vi "UHR-Fleezers Control (host) -Leonardo 04-2018 V4_fish.vi"(0 "Tab Green FB":T5(tab)=enum."Trap Control (RF)") -> ()   [LabVIEW 2014] (continued)
          tunnel: [w3580 w3581] -> w3547
          frame False {
          }
          frame True {
            n1861 = Array Subset(array=w3586, index (row)=0 ("index"), length (row)=4 ("length"), index (col)=0 ("index"), length (col)=1 ("length")) -> (w3581:T47)
          }
        }
        n1862 = feedback-in #9(w3547) -> ()
        n1863 = Split 1D Array(array=w3561, index=2) -> (first subarray=→"FFT 1":cluster{"f0":dbl, "df":dbl, "magnitude":dbl[]}[], second subarray=→"FFT 2":cluster{"f0":dbl, "df":dbl, "magnitude":dbl[]}[])
      }
    }
    n1864 = Index Array(array=w2395, index=1) -> (element=w2403:waveform(dbl))
    n1865 = case "For displaying the high resolution display (no downsampling)" shown="True" w2459 {
      tunnel: w2422 -> [_ w2789]
      frame False {
      }
      frame True {
        n1866 = Index Array(array=w2789, index="High Res. Display") -> (element=w2790:waveform(dbl))
        n1867 = call <vilib>:"Std Deviation and Variance.vi"("X"=w2790) -> ("mean"=w2797:dbl, "standard deviation"=w2802:dbl)  [unwired: 1 in, 1 out]
        "Mean Intensity" <- w2797
        "Sigma" <- w2802
        n1868 = Subtract(x=w2790, y=w2797) -> (x-y=w2796:waveform(dbl))
        n1869 = Select(t=w2796, s="Subtract mean", f=w2790) -> (s? t:f=→"1 Channel":waveform(dbl))
        n1870 = Divide(x=w2802, y=w2797) -> (x/y=→"Sigma/Mean":dbl)
        n1871 = feedback #10(1) -> (w2791:i32)
        n1872 = Greater Or Equal?(x=w2791, y="Slow mean N ave.") -> (x >= y?=w2804:bool)
        n1873 = Increment(x=w2791) -> (x+1=w2806:i32)
        n1874 = Select(t=1, s=w2804, f=w2806) -> (s? t:f=w2793:i32)
        n1875 = feedback-in #10(w2793) -> ()
        n1876 = feedback #11() -> (w2794:waveform(dbl))  [unwired: 1 out]
        n1877 = case shown="Default" w2791 {
          tunnel: [w2809 w2812] -> w2795
          tunnel: w2794 -> [w2811 _]
          tunnel: w2790 -> [w2810 w2812]
          frame Default {
            n1878 = call-poly <vilib>:"Append Waveforms.vi"("waveform B"=w2810, "waveform A"=w2811) -> ("waveform out"=w2809:waveform(dbl))  [unwired: 1 in, 8 out]
          }
          frame 1 {
          }
        }
        n1879 = feedback-in #11(w2795) -> ()
        n1880 = case shown="True" w2804 {
          tunnel: w2795 -> [_ w2808]
          frame False {
          }
          frame True {
            n1881 = call-poly <vilib>:"Mean.vi"("X"=w2808) -> ("mean"=→"Slow mean":dbl)  [unwired: 1 out]
          }
        }
      }
    }
    n1882 = case "For plotting results of scanning MCL" shown="True" w2529 {
      tunnel: w2528 -> [_ w2929]
      tunnel: w2452 -> [_ w3025]
      tunnel: w2537 -> [_ _]
      tunnel: w2422 -> [_ w2999]
      tunnel: w2397 -> [_ w2930]
      tunnel: w2396 -> [_ w2903]
      frame False {
      }
      frame True {
        w2910 = u32 0 items=["Horizontal", "Vertical", "Central", "1st Diagonal", "2nd Diagonal"] ("Type of Symmetry")
        w2938 = u32 0 items=["Horizontal", "Vertical", "Central", "1st Diagonal", "2nd Diagonal"] ("Type of Symmetry")
        w2941 = u32 0 items=["Horizontal", "Vertical", "Central", "1st Diagonal", "2nd Diagonal"] ("Type of Symmetry")
        w2970 = u32 0 items=["Horizontal", "Vertical", "Central", "1st Diagonal", "2nd Diagonal"] ("Type of Symmetry")
        n1883 = Index Array(array=w2999, index=10) -> (element=w3005:waveform(dbl))
        n1884 = Index Array(array=w2999, index=11) -> (element=w3002:waveform(dbl))
        n1885 = local read "Cycles/step (MCL)"() -> (w2955:u64)
        n1886 = Index Array(array=w2999, index="Channel") -> (element=w3001:waveform(dbl))
        n1887 = Unbundle(w2903) -> ("New Image"=w2902:T3, "New Image"=w2901:T3, "New Image"=w2900:T3, "New Image"=w2899:T3)
        n1888 = Unbundle By Name(w3005) -> ("Y"=w2957:dbl[])
        n1889 = Unbundle By Name(w3002) -> ("Y"=w2959:dbl[])
        n1890 = Unbundle By Name(w3001) -> ("Y"=w2964:dbl[])
        n1891 = call "downsample 1D array - double.vi"("Ave N"=w2955, "Array In"=w2957) -> ("Array Out"=w2956:dbl[])  [unwired: 1 out]
        n1892 = call "downsample 1D array - double.vi"("Ave N"=w2955, "Array In"=w2959) -> ("Array Out"=w2958:dbl[])  [unwired: 1 out]
        n1893 = call "downsample 1D array - double.vi"("Ave N"=w2955, "Array In"=w2964) -> ("Array Out"=w2963:dbl[])  [unwired: 1 out]
        n1894 = feedback #12(w3025) -> (w3026:dbl[])
        n1895 = Build Array (concatenate)(w3026, w3025) -> (w3007:dbl[])
        n1896 = feedback #13(w2930) -> (w2932:dbl[])
        n1897 = Build Array (concatenate)(w2932, w2930) -> (w2931:dbl[])
        n1898 = local read "Scan steps (MCL)"() -> (w2912:u64)
        n1899 = Select(t=w3025, s=w2929, f=w3007) -> (s? t:f=w3011:dbl[])
        n1900 = feedback-in #12(w3011) -> ()
        n1901 = Select(t=w2930, s=w2929, f=w2931) -> (s? t:f=w2913:dbl[])
        n1902 = feedback-in #13(w2913) -> ()
        n1903 = local read "Scan lines (y)"() -> (w2898:u64)
        n1904 = local read "N APD Samp/step"() -> (w2914:dbl)
        n1905 = feedback #14(w2956) -> (w3013:dbl[])
        n1906 = Build Array (concatenate)(w3013, w2956) -> (w3004:dbl[])
        n1907 = feedback #15(w2963) -> (w3023:dbl[])
        n1908 = Build Array (concatenate)(w3023, w2963) -> (w3022:dbl[])
        n1909 = feedback #16(w2958) -> (w3015:dbl[])
        n1910 = Build Array (concatenate)(w3015, w2958) -> (w3016:dbl[])
        n1911 = Select(t=w2956, s=w2929, f=w3004) -> (s? t:f=w2960:dbl[])
        n1912 = feedback-in #14(w2960) -> ()
        n1913 = Select(t=w2963, s=w2929, f=w3022) -> (s? t:f=w2962:dbl[])
        n1914 = feedback-in #15(w2962) -> ()
        n1915 = Select(t=w2958, s=w2929, f=w3016) -> (s? t:f=w2961:dbl[])
        n1916 = feedback-in #16(w2961) -> ()
        n1917 = Multiply(x=w2912, y=u64 2) -> (x*y=w2897:u64)
        n1918 = call "integrate 1D array interval - double.vi"("Ave N"=w2914, "Array In"=w2913) -> ("Array Out"=w2925:dbl[])  [unwired: 1 out]
        n1919 = call "integrate 1D array interval - double.vi"("Ave N"=w2914, "Array In"=w3011) -> ("Array Out"=w3010:dbl[])  [unwired: 1 out]
        n1920 = Array Size(array=w2925) -> (size(s)=w2926:i32)
        n1921 = Array Size(array=w3010) -> (size(s)=w3012:i32)
        n1922 = Multiply(x=w2898, y=w2897) -> (x*y=w2928:u64)
        n1923 = Multiply(x=w2898, y=w2897) -> (x*y=w3020:u64)
        n1924 = call-poly <vilib>:"Mean.vi"("X"=w2960) -> ("mean"=w2944:dbl)  [unwired: 1 out]
        n1925 = Subtract(x=w2928, y=w2926) -> (x-y=w2919:u64)
        n1926 = call-poly <vilib>:"Mean.vi"("X"=w2962) -> ("mean"=w2949:dbl)  [unwired: 1 out]
        n1927 = call-poly <vilib>:"Mean.vi"("X"=w2961) -> ("mean"=w2947:dbl)  [unwired: 1 out]
        n1928 = call-poly <vilib>:"Mean.vi"("X"=w2925) -> ("mean"=w2916:dbl)  [unwired: 1 out]
        n1929 = Subtract(x=w3020, y=w3012) -> (x-y=w2954:u64)
        n1930 = call-poly <vilib>:"Mean.vi"("X"=w3010) -> ("mean"=w2951:dbl)  [unwired: 1 out]
        n1931 = Initialize Array(1.0 ("element"), w2919) -> (w2915:dbl[])
        n1932 = Initialize Array(1.0 ("element"), w2954) -> (w2945:dbl[])
        n1933 = Multiply(x=w2915, y=w2916) -> (x*y=w2917:dbl[])
        n1934 = Multiply(x=w2945, y=w2947) -> (x*y=w2948:dbl[])
        n1935 = Multiply(x=w2945, y=w2949) -> (x*y=w2950:dbl[])
        n1936 = Multiply(x=w2945, y=w2944) -> (x*y=w2946:dbl[])
        n1937 = Multiply(x=w2945, y=w2951) -> (x*y=w2952:dbl[])
        n1938 = Build Array (concatenate)(w2960, w2946) -> (w3014:dbl[])
        n1939 = Build Array (concatenate)(w2962, w2950) -> (w3018:dbl[])
        n1940 = Build Array (concatenate)(w2961, w2948) -> (w3017:dbl[])
        n1941 = Build Array (concatenate)(w2925, w2917) -> (w2927:dbl[])
        n1942 = Build Array (concatenate)(w3010, w2952) -> (w3019:dbl[])
        n1943 = Reshape Array(w3014, w2898, w2897) -> (w2980:dbl[][])
        n1944 = Reshape Array(w2927, w2898, w2897) -> (w2923:dbl[][])
        n1945 = Reshape Array(w3018, w2898, w2897) -> (w2972:dbl[][])
        n1946 = Reshape Array(w3017, w2898, w2897) -> (w2987:dbl[][])
        n1947 = Reshape Array(w3019, w2898, w2897) -> (w2997:dbl[][])
        n1948 = Array Subset(array=w2987, index (col)=0 ("index"), length (col)=w2912) -> (w2992:dbl[][])  [unwired: 2 in]
        n1949 = Array Subset(array=w2987, index (col)=w2912) -> (w2990:dbl[][])  [unwired: 3 in]
        n1950 = Array Subset(array=w2972, index (col)=0 ("index"), length (col)=w2912) -> (w2978:dbl[][])  [unwired: 2 in]
        n1951 = Array Subset(array=w2972, index (col)=w2912) -> (w2976:dbl[][])  [unwired: 3 in]
        n1952 = Array Subset(array=w2923, index (col)=0 ("index"), length (col)=w2912) -> (w2922:dbl[][])  [unwired: 2 in]
        n1953 = Array Subset(array=w2923, index (col)=w2912) -> (w2920:dbl[][])  [unwired: 3 in]
        n1954 = Array Subset(array=w2997, index (col)=0 ("index"), length (col)=w2912) -> (w2996:dbl[][])  [unwired: 2 in]
        n1955 = Array Subset(array=w2997, index (col)=w2912) -> (w2994:dbl[][])  [unwired: 3 in]
        n1956 = Array Subset(array=w2980, index (col)=0 ("index"), length (col)=w2912) -> (w2985:dbl[][])  [unwired: 2 in]
        n1957 = Array Subset(array=w2980, index (col)=w2912) -> (w2983:dbl[][])  [unwired: 3 in]
        n1958 = for {
          tunnel: w2992 -> [w3034] mode=indexing
          tunnel: [w3033] -> w2991 mode=indexing
          workers-P: _ -> [_]
          n1959 = Reverse 1D Array(array=w3034) -> (reversed array=w3033:dbl[])
        }
        n1960 = for {
          tunnel: w2978 -> [w3030] mode=indexing
          tunnel: [w3029] -> w2977 mode=indexing
          workers-P: _ -> [_]
          n1961 = Reverse 1D Array(array=w3030) -> (reversed array=w3029:dbl[])
        }
        n1962 = for {
          tunnel: w2922 -> [w3028] mode=indexing
          tunnel: [w3027] -> w2921 mode=indexing
          workers-P: _ -> [_]
          n1963 = Reverse 1D Array(array=w3028) -> (reversed array=w3027:dbl[])
        }
        n1964 = for {
          tunnel: w2996 -> [w3036] mode=indexing
          tunnel: [w3035] -> w2995 mode=indexing
          workers-P: _ -> [_]
          n1965 = Reverse 1D Array(array=w3036) -> (reversed array=w3035:dbl[])
        }
        n1966 = for {
          tunnel: w2985 -> [w3032] mode=indexing
          tunnel: [w3031] -> w2984 mode=indexing
          workers-P: _ -> [_]
          n1967 = Reverse 1D Array(array=w3032) -> (reversed array=w3031:dbl[])
        }
        n1968 = Index Array(array=w2997, index (row)=0) -> (element=→"Waveform Graph":dbl[])  [unwired: 1 in]
        n1969 = Add(x=w2991, y=w2990) -> (x+y=w2989:dbl[][])
        n1970 = Add(x=w2977, y=w2976) -> (x+y=w2975:dbl[][])
        n1971 = Add(x=w2921, y=w2920) -> (x+y=w2905:dbl[][])
        n1972 = Add(x=w2995, y=w2994) -> (x+y=w2969:dbl[][])
        n1973 = Add(x=w2984, y=w2983) -> (x+y=w2982:dbl[][])
        n1974 = Divide(x=w2975, y=2) -> (x/y=w2973:dbl[][])
        n1975 = Divide(x=w2989, y=2) -> (x/y=w2934:dbl[][])
        n1976 = Divide(x=w2982, y=2) -> (x/y=w2936:dbl[][])
        n1977 = To Single Precision Float(number=w2969) -> (single precision float=w2968:sgl[][])
        n1978 = Transpose 2D Array(2D array=w2973) -> (transposed array=→"Data map":dbl[][])
        n1979 = To Single Precision Float(number=w2905) -> (single precision float=w2909:sgl[][])
        n1980 = To Single Precision Float(number=w2934) -> (single precision float=w2940:sgl[][])
        n1981 = To Single Precision Float(number=w2936) -> (single precision float=w2937:sgl[][])
        n1982 = call "IMAQ ArrayToImage"("Image Pixels (Float)"=w2968, "Image"=w2902) -> ("Image Out"=w2971:T3)  [unwired: 8 in, 1 out]
        n1983 = call "IMAQ ArrayToImage"("Image Pixels (Float)"=w2909, "Image"=w2901) -> ("Image Out"=w2911:T3)  [unwired: 8 in, 1 out]
        n1984 = call "IMAQ ArrayToImage"("Image Pixels (Float)"=w2940, "Image"=w2900) -> ("Image Out"=w2942:T3)  [unwired: 8 in, 1 out]
        n1985 = call "IMAQ ArrayToImage"("Image Pixels (Float)"=w2937, "Image"=w2899) -> ("Image Out"=w2939:T3)  [unwired: 8 in, 1 out]
        n1986 = call "IMAQ Symmetry"("Type of Symmetry"=w2970, "Image Src"=w2971) -> ("Image Dst Out"=w2966:T3)  [unwired: 3 in, 1 out]
        n1987 = call "IMAQ Symmetry"("Type of Symmetry"=w2910, "Image Src"=w2911) -> ("Image Dst Out"=w2907:T3)  [unwired: 3 in, 1 out]
        n1988 = call "IMAQ Symmetry"("Type of Symmetry"=w2941, "Image Src"=w2942) -> ("Image Dst Out"=→"Detection Laser X":T3)  [unwired: 3 in, 1 out]
        n1989 = call "IMAQ Symmetry"("Type of Symmetry"=w2938, "Image Src"=w2939) -> ("Image Dst Out"=→"Detection Laser Y":T3)  [unwired: 3 in, 1 out]
        n1990 = call "IMAQ Set Simple Calibration"("Calibration Axis Info"=T37 {"Origin Pixel"={"X"=0.0, "Y"=0.0}, "Angle Relative to Horizontal (deg)"=0.0, "Axis Reference"=0}, "Grid Descriptor"=T38 {"X Step"=0.3, "Y Step"=0.3, "Unit"=enum."Undefined"}, "Image"=w2966) -> ("Calibrated Image"=→"APD 1":T3)  [unwired: 7 in, 1 out]
        n1991 = call "IMAQ Set Simple Calibration"("Calibration Axis Info"=T37 {"Origin Pixel"={"X"=0.0, "Y"=0.0}, "Angle Relative to Horizontal (deg)"=0.0, "Axis Reference"=0}, "Grid Descriptor"=T38 {"X Step"=0.3, "Y Step"=0.3, "Unit"=enum."Undefined"}, "Image"=w2907) -> ("Calibrated Image"=→"APD 2":T3)  [unwired: 7 in, 1 out]
      }
    }
    n1992 = Subtract(x=w2403, y="APD 2 Offset") -> (x-y=w2400:waveform(dbl))
    n1993 = Subtract(x=w2405, y="APD 1 Offset") -> (x-y=w2401:waveform(dbl))
    n1994 = Index Array(array=w2420, index=3) -> (element=w2479:waveform(dbl))
    n1995 = Index Array(array=w2420, index=6) -> (element=w2476:waveform(dbl))
    n1996 = Build Array(w2401, w2400) -> (→"APD Chart":waveform(dbl)[])
    n1997 = Array Size(array=w2469) -> (size(s)=w2517:i32)
    n1998 = call <vilib>:"Std Deviation and Variance.vi"("X"=w2413) -> ("standard deviation"=w2412:dbl)  [unwired: 1 in, 2 out]
    n1999 = Add Array Elements(numeric array=w2413) -> (sum=w2415:u32)
    n2000 = Add Array Elements(numeric array=w2469) -> (sum=w2527:u32)
    n2001 = call <vilib>:"Std Deviation and Variance.vi"("X"=w2469) -> ("standard deviation"=w2468:dbl)  [unwired: 1 in, 2 out]
    n2002 = Divide(x=w2412, y=w2411) -> (x/y=w2408:dbl)
    "Rate sigma (Hz) 2" <- w2408
    n2003 = Multiply(x=w2411, y=w2517) -> (x*y=w2414:dbl)
    "Int. Time (s)" <- w2414
    n2004 = Divide(x=w2415, y=w2414) -> (x/y=w2409:dbl)
    "APD 2 Rate (Hz)" <- w2409
    n2005 = Divide(x=w2527, y=w2414) -> (x/y=w2466:dbl)
    "APD 1 Rate (Hz)" <- w2466
    n2006 = Divide(x=w2468, y=w2411) -> (x/y=w2467:dbl)
    "Rate sigma (Hz)" <- w2467
    n2007 = Divide(x=w2408, y=w2409) -> (x/y=→"Sigma/Mean 2":dbl)
    n2008 = Divide(x=w2467, y=w2466) -> (x/y=→"Sigma/Mean":dbl)
    n2009 = case shown="2" "Calibration" {
      tunnel: "T1 alpha_x (nm/V)" -> [_ w2865 w2886]
      tunnel: "T1 kappa_x (pN/nm)" -> [_ _ w2876]
      tunnel: "T2 alpha_x (nm/V)" -> [_ w2864 w2884]
      tunnel: "T2 kappa_x (pN/nm)" -> [_ _ w2877]
      tunnel: w2479 -> [w2847 w2862 w2882]
      tunnel: w2476 -> [w2846 w2860 w2880]
      tunnel: [w2847 w2859 w2879] -> w2270
      tunnel: [w2846 w2858 w2878] -> w2276
      tunnel: ["T1 X (V)" ("Label.Text") "T1 X (nm)" ("Label.Text") "T1 X (pN)" ("Label.Text")] -> w2497
      tunnel: ["T2 X (V)" ("Label.Text") "T2 X (nm)" ("Label.Text") "T2 X (pN)" ("Label.Text")] -> w2496
      tunnel: ["Position (V)" ("Label.Text") "Position (nm)" ("Label.Text") "Force (pN)" ("Label.Text")] -> w2498
      tunnel: w2478 -> [_ w2850 w2869]
      tunnel: w2480 -> [_ w2853 w2871]
      tunnel: ["Mean (V)" ("Label.Text") "Mean (nm)" ("Label.Text") "Mean (pN)" ("Label.Text")] -> w2493
      tunnel: ["Difference (V)" ("Label.Text") "Difference (nm)" ("Label.Text") "Difference (pN)" ("Label.Text")] -> w2428
      frame 0, Default {
      }
      frame 1 {
        # "position"
        n2010 = Unbundle By Name(w2862) -> ("Y"=w2866:dbl[])
        n2011 = Unbundle By Name(w2860) -> ("Y"=w2851:dbl[])
        n2012 = Subtract(x=w2866, y=w2853) -> (x-y=w2854:dbl[])
        n2013 = Subtract(x=w2851, y=w2850) -> (x-y=w2852:dbl[])
        n2014 = Multiply(x=w2852, y=w2864) -> (x*y=w2861:dbl[])
        n2015 = Multiply(x=w2865, y=w2854) -> (x*y=w2863:dbl[])
        n2016 = Bundle By Name(cluster=w2860, "Y"=w2861) -> (w2858:waveform(dbl))
        n2017 = Bundle By Name(cluster=w2862, "Y"=w2863) -> (w2859:waveform(dbl))
      }
      frame 2 {
        # "force"
        n2018 = Unbundle By Name(w2882) -> ("Y"=w2887:dbl[])
        n2019 = Unbundle By Name(w2880) -> ("Y"=w2885:dbl[])
        n2020 = Subtract(x=w2885, y=w2869) -> (x-y=w2870:dbl[])
        n2021 = Subtract(x=w2887, y=w2871) -> (x-y=w2872:dbl[])
        n2022 = Compound Arithmetic op=MULTIPLY(w2870, w2884, w2877) -> (w2881:dbl[])
        n2023 = Compound Arithmetic op=MULTIPLY(w2876, w2886, w2872) -> (w2883:dbl[])
        n2024 = Bundle By Name(cluster=w2880, "Y"=w2881) -> (w2878:waveform(dbl))
        n2025 = Bundle By Name(cluster=w2882, "Y"=w2883) -> (w2879:waveform(dbl))
      }
    }
    n2026 = feedback-in #17("Calibration") -> ()
    n2027 = feedback #17(u16 1 ("Calibration")) -> (w2500:u16)
    n2028 = local read "Trap 2 Bead Size (nm)"() -> (w2308:dbl)
    n2029 = local read "Trap 1 Bead Size (nm)"() -> (w2307:dbl)
    n2030 = local read "AOM X Cal (nm/MHz)"() -> (w2305:dbl)
    n2031 = local read "Trap Delta (MHz)"() -> (w2304:dbl)
    n2032 = Not Equal?(x=w2500, y="Calibration") -> (x != y?=w2457:bool)
    n2033 = Multiply(x=w2305, y=w2304) -> (x*y=w2309:dbl)
    n2034 = Unbundle By Name(w2270) -> ("Y"=w2275:dbl[])
    n2035 = Unbundle By Name(w2276) -> ("Y"=w2274:dbl[])
    n2036 = Add(x=w2308, y=w2307) -> (x+y=w2311:dbl)
    n2037 = case shown="False" "Negate trap 2 force" {
      tunnel: [-1.0 1.0] -> w2486
      frame False {
      }
      frame True {
      }
    }
    n2038 = Unbundle By Name(w2479) -> ("Y"=w2482:dbl[])
    n2039 = Unbundle By Name(w2476) -> ("Y"=w2485:dbl[])
    n2040 = Divide(x=w2311, y=2.0) -> (x/y=w2306:dbl)
    n2041 = Subtract(x=w2275, y=w2274) -> (x-y=w2272:dbl[])
    n2042 = Subtract(x=w2482, y=w2480) -> (x-y=w2483:dbl[])
    n2043 = Subtract(x=w2485, y=w2478) -> (x-y=w2484:dbl[])
    n2044 = Divide(x=w2272, y=2.0) -> (x/y=w2271:dbl[])
    n2045 = Multiply(x=w2484, y="T2 alpha_x (nm/V)") -> (x*y=w2475:dbl[])
    n2046 = Multiply(x="T1 alpha_x (nm/V)", y=w2483) -> (x*y=w2474:dbl[])
    n2047 = Multiply(x=w2276, y=w2486) -> (x*y=w2487:waveform(dbl))
    n2048 = Bundle By Name(cluster=w2270, "Y"=w2271) -> (w2269:waveform(dbl))
    n2049 = case shown="True" "Read Lateness and Rel Phase" {
      tunnel: w2281 -> [w2813 w2835]
      tunnel: w2320 -> [w2814 w2834]
      tunnel: [w2813 w2833] -> w2472
      tunnel: [w2814 w2832] -> w2471
      frame False {
      }
      frame True {
        n2050 = xnode "Read/Write Control"("FPGA VI Reference In"=w2835, "error in"=w2834) -> ("FPGA VI Reference Out"=w2833:T20, "error out"=w2832:errorcluster, "GI Relative phase"=→"GI relative phase":i16, "Relative phase"=→"Relative phase (AI1)":i16, "AI Late Counter"=→"Late Counter (AI1)":u8, "GI Late Counter"=→"GI Late Counter":u8, "MCL Late Counter"=→"MCL Late Counter":u8, "MCL Relative Phase"=→"Relative Phase (MCL)":i16, "APD Acq Relative Phase"=→"APD Acq Relative Phase":i16, "APD 1 Gate Relative Phase"=→"APD 1 Gate Relative Phase":i16, "APD 2 Gate Relative Phase"=→"APD 2 Gate Relative Phase":i16, "APD Acq Late Counter"=→"APD Acq Late Counter":u16, "APD 1 Gate Late Counter"=→"APD 1 Gate Late Counter":u8, "APD 2 Gate Late Counter"=→"APD 2 Gate Late Counter":u8, "Green FB Relative Phase"=→"Relative phase (Green FB)":i16, "GI Relative phase"=→"GI relative phase 2":i16, "GI Late Counter 2"=→"GI Late Counter 2":u16, "Trap Pos FIFO Timeout"=→"Trap Pos FIFO Timeout":u16, "Trap AI FIFO Timeout"=→"Trap AI FIFO Timeout":u16)
      }
    }
    n2051 = Subtract(x=w2475, y=w2474) -> (x-y=w2303:dbl[])
    n2052 = call-poly <vilib>:"Mean.vi"("X"=w2303) -> ("mean"=w2310:dbl)  [unwired: 1 out]
    n2053 = Add(x=w2309, y=w2310) -> (x+y=w2313:dbl)
    n2054 = Subtract(x=w2313, y=w2306) -> (x-y=→"Tether Extension (nm, calculated)":dbl)
    n2055 = Unbundle By Name(w2276) -> ("Y"=w2267:dbl[])
    n2056 = Unbundle By Name(w2270) -> ("Y"=w2268:dbl[])
    n2057 = Build Array(w2270, w2487, w2269) -> (→"Force":waveform(dbl)[])
    n2058 = Subtract(x=w2303, y="Offset (nm)") -> (x-y=w2447:dbl[])
    n2059 = call-poly <vilib>:"Mean.vi"("X"=w2267) -> ("mean"=w2265:dbl)  [unwired: 1 out]
    "T2 X" <- w2265
    n2060 = call-poly <vilib>:"Mean.vi"("X"=w2268) -> ("mean"=w2266:dbl)  [unwired: 1 out]
    "T1 X" <- w2266
    n2061 = Subtract(x=w2268, y=w2267) -> (x-y=w2449:dbl[])
    n2062 = Bundle By Name(cluster=w2479, "Y"=w2447) -> (w2419:waveform(dbl))
    "Bead Separation" <- w2419
    n2063 = Divide(x=w2449, y=2.0) -> (x/y=→"Vec Mean of T1 T2":dbl[])
    n2064 = case shown="True" w2457 {
      tunnel: w2498 -> [_ w2840]
      tunnel: w2497 -> [_ w2839]
      tunnel: w2496 -> [_ w2838]
      tunnel: w2493 -> [_ w2837]
      tunnel: w2428 -> [_ w2836]
      frame False {
      }
      frame True {
        n2065 = property on="Force" class="WFChart (strict)"("YScale.NameLbl.Text"=w2840) -> ()  [unwired: 2 in, 2 out]
        n2066 = property on="T2 X" class="DigNum (strict)"("Caption.Text"=w2838) -> ()  [unwired: 2 in, 2 out]
        n2067 = property on="T1 X" class="DigNum (strict)"("Caption.Text"=w2839) -> ()  [unwired: 2 in, 2 out]
        n2068 = property on="Mean" class="DigNum (strict)"("Caption.Text"=w2837) -> ()  [unwired: 2 in, 2 out]
        n2069 = property on="Difference" class="DigNum (strict)"("Caption.Text"=w2836) -> ()  [unwired: 2 in, 2 out]
      }
    }
    n2070 = local read "Tether"() -> (w2451:bool)
    n2071 = Subtract(x=w2266, y=w2265) -> (x-y=w2495:dbl)
    n2072 = Add(x=w2266, y=w2265) -> (x+y=→"Difference":dbl)
    n2073 = feedback #18(w2447) -> (w2446:dbl[])
    n2074 = Divide(x=w2495, y=2.0) -> (x/y=w2245:dbl)
    "Mean" <- w2245
    n2075 = case shown="True" w2451 {
      tunnel: w2245 -> [_ w2772]
      frame False {
      }
      frame True {
        n2076 = Greater?(x="Lost Tether Alarm Threshold (pN)", y=w2772) -> (0:w2770:bool)
        n2077 = case shown="True" w2770 {
          frame False {
          }
          frame True {
            n2078 = flat-sequence {
              frame #0 {
                # "stop only if saving"
                n2079 = local read "Saving..."() -> (w2785:bool)
                n2080 = And(x=w2785, y="TA Cancel Save?") -> (x .and. y?=w2784:bool)
                n2081 = local write "Stop Saving"(w2784) -> ()
              }
              frame #1 {
                n2082 = case shown="True" "TA Green Off?" {
                  frame False {
                  }
                  frame True {
                    w2788 = FALSE ("Fl. Triggered...")
                    n2083 = local write "Fl. Triggered..."(w2788) -> ()
                    n2084 = property on="Green Laser ON/Interlacing" class="Bool (strict)"("Val(Sgnl)"=w2788) -> ()  [unwired: 2 in, 2 out]
                  }
                }
              }
            }
            n2085 = local read "Time tether formed"() -> (w2779:timestamp)
            n2086 = Get Date/Time In Seconds() -> (seconds since 1Jan1904=w2780:timestamp)
            n2087 = Subtract(x=w2780, y=w2779) -> (x-y=w2778:dbl)
            n2088 = Number To Decimal String(number=w2778) -> (decimal integer string=w2775:string)  [unwired: 1 out]
            n2089 = local read "Messages"() -> (w2782:string)
            n2090 = call <vilib>:"Beep.vi"() -> ()  [unwired: 3 in, 9 out]
            n2091 = Concatenate Strings("Lost tether (" ("Message to add"), w2775, " s)." ("string")) -> (w2777:string)
            n2092 = local write "Tether"(FALSE ("Tether")) -> ()
            n2093 = call "Update messages.vi"("Message to add"=w2777, "Old message string"=w2782) -> ("New message string"=w2781:string)
            n2094 = local write "Messages"(w2781) -> ()
            n2095 = property on="Trap Pos. FB ON" class="Bool (strict)"("Val(Sgnl)"=FALSE ("Value (Signaling)")) -> ()  [unwired: 2 in, 2 out]
          }
        }
      }
    }
    n2096 = Build Array (concatenate)(w2447, w2446) -> (w2445:dbl[])
    n2097 = Split 1D Array(array=w2445, index=w2331) -> (first subarray=w2441:dbl[])  [unwired: 1 out]
    n2098 = feedback-in #18(w2441) -> ()
    n2099 = call-poly <vilib>:"Mean.vi"("X"=w2441) -> ("mean"=w2440:dbl)  [unwired: 1 out]
    "Bead Mean (nm)" <- w2440
    n2100 = Subtract(x=w2441, y=w2440) -> (x-y=w2439:dbl[])
    n2101 = Square(x=w2439) -> (x^2=w2438:dbl[])
    n2102 = case shown="True" "Semi Passive ON" {
      tunnel: "Semi Passive mode" -> [_ w2653]
      tunnel: "Jump Force (pN)" -> [_ w2652]
      tunnel: w2245 -> [_ w2651]
      frame False {
      }
      frame True {
        n2103 = case shown="\"Sharp Jump\"" w2653 {
          tunnel: w2652 -> [_ w2656 w2672]
          tunnel: w2651 -> [_ w2655 w2671]
          frame "None" {
          }
          frame "Use Feedback" {
            n2104 = local read "Target Force (pN)"() -> (w2658:dbl)
            n2105 = Less?(x=w2656, y=w2658) -> (x < y?=w2657:bool)
            n2106 = case shown="True" w2657 {
              tunnel: w2656 -> [w2665 w2668]
              tunnel: w2655 -> [w2664 w2667]
              tunnel: [w2663 w2666] -> w2654
              frame False {
                n2107 = Less?(x=w2665, y=w2664) -> (x < y?=w2663:bool)
              }
              frame True {
                n2108 = Greater?(x=w2668, y=w2667) -> (0:w2666:bool)
              }
            }
            n2109 = case shown="True" w2654 {
              frame False {
                n2110 = local read "Trap Pos. FB ON"() -> (w2659:bool)
                n2111 = case shown="True" w2659 {
                  frame False {
                  }
                  frame True {
                    n2112 = property on="Trap Pos. FB ON" class="Bool (strict)"("Val(Sgnl)"=FALSE) -> ()  [unwired: 2 in, 2 out]
                  }
                }
              }
              frame True {
                n2113 = local read "Trap Pos. FB ON"() -> (w2661:bool)
                n2114 = case shown="False" w2661 {
                  frame False {
                    n2115 = property on="Trap Pos. FB ON" class="Bool (strict)"("Val(Sgnl)"=TRUE) -> ()  [unwired: 2 in, 2 out]
                  }
                  frame True {
                  }
                }
              }
            }
          }
          frame "Sharp Jump" {
            n2116 = local read "Target Force (pN)"() -> (w2674:dbl)
            n2117 = Greater?(x=w2672, y=w2674) -> (0:w2673:bool)
            n2118 = case shown="True" w2673 {
              tunnel: w2672 -> [w2689 w2693]
              tunnel: w2671 -> [w2690 w2692]
              tunnel: [w2688 w2691] -> w2670
              frame False {
                n2119 = Greater?(x=w2690, y=w2689) -> (0:w2688:bool)
              }
              frame True {
                n2120 = Less?(x=w2693, y=w2692) -> (x < y?=w2691:bool)
              }
            }
            n2121 = Subtract(x=w2672, y=w2674) -> (x-y=w2669:dbl)
            n2122 = case shown="True" w2670 {
              tunnel: w2669 -> [_ w2680]
              frame False {
              }
              frame True {
                n2123 = local read "T1 kappa_x (pN/nm)"() -> (w2685:dbl)
                n2124 = local read "T2 kappa_x (pN/nm)"() -> (w2686:dbl)
                n2125 = Reciprocal(x="DNA stiffness (pN / nm)") -> (1/x=w2682:dbl)
                n2126 = Reciprocal(x=w2685) -> (1/x=w2684:dbl)
                n2127 = Reciprocal(x=w2686) -> (1/x=w2683:dbl)
                n2128 = Compound Arithmetic op=ADD(w2684, w2683, w2682) -> (w2681:dbl)
                n2129 = local read "AOM X Cal (nm/MHz)"() -> (w2679:dbl)
                n2130 = Multiply(x=w2681, y=w2680) -> (x*y=w2678:dbl)
                n2131 = local read "Trap Delta (MHz)"() -> (w2676:dbl)
                n2132 = Divide(x=w2678, y=w2679) -> (x/y=w2677:dbl)
                n2133 = Subtract(x=w2676, y=w2677) -> (x-y=w2675:dbl)
                n2134 = property on="Trap Delta (MHz)" class="DigNum (strict)"("Val(Sgnl)"=w2675) -> ()  [unwired: 2 in, 2 out]
              }
            }
          }
        }
      }
    }
    n2135 = call-poly <vilib>:"Mean.vi"("X"=w2438) -> ("mean"=w2437:dbl)  [unwired: 1 out]
    n2136 = Square Root(x=w2437) -> (sqrt(x)=w2436:dbl)
    n2137 = Multiply(x=10.0, y=w2436) -> (x*y=→"RMS (Ang)":dbl)
    n2138 = xnode "Read/Write Control"("FPGA VI Reference In"=w2472, "error in"=w2471) -> ("FPGA VI Reference Out"=w2581:T20, "error out"=w2575:errorcluster, "AI2 Y Sum Set 1"=w2571:i16, "AI2 Y Sum Set 2"=w2570:i16, "AI1 X Set 1"=w2365:fxp<+/-,16,1>, "AI1 X Set 2"=w2364:fxp<+/-,16,1>, "Trap Pos FB Int Signal"=→"Trap Pos FB Int Signal":fxp<+/-,24,9>, "Trap Pos FB Int-Norm Signal"=→"Trap Pos FB Int-Norm Signal":fxp<+/-,16,1>, "Trap Pos FB Action"=w2358:i64, "Scanning"=→"AOD Scanning":bool, "Scan I"=→"AOD Scan I":u64, "Scanning MCL"=w2573:bool, "Scan I (MCL)"=→"MCL Scan I":u64, "Green FB Signals"=w2512:T48, "BD1 amplitude 1 out"=w2264:u16, "BD1 amplitude 2 out"=w2249:u16)  [unwired: 1 out]
    "MCL Scanning" <- w2573
    "Trap Pos FB Action" <- w2358
    n2139 = local read "Fish Status"() -> (w2244:u16)
    n2140 = local read "AI2 (V)"() -> (w2572:cluster{"Set 1":dbl, "Set 2":dbl})
    n2141 = case shown="False" "Toggle AFish" {
      tunnel: w2245 -> [w2594 _]
      tunnel: w2244 -> [w2593 w2637]
      frame False {
        n2142 = case "Autofishing - Alex" shown="4" w2593 {
          tunnel: w2594 -> [_ _ _ w2623 _]
          frame 0, Default {
            # "Off"
          }
          frame 1 {
            # "Approach"
            n2143 = local read "Trap Delta (MHz)"() -> (w2597:dbl)
            n2144 = Add(x=w2597, y="Approach dTD") -> (x+y=w2596:dbl)
            n2145 = In Range and Coerce(upper limit=inf, x=w2596, lower limit="Min TD") -> (coerced(x)=w2598:dbl, In Range?=w2599:bool)
            n2146 = case shown="False" w2599 {
              frame False {
                w2603 = u16 2 items=["Off", "Approach", "Wiggle", "Extend", "Tether Found"] ("Fish Status")
                n2147 = Tick Count (ms)() -> (millisecond timer value=→"AF Time":u32)
                n2148 = local write "Fish Status"(w2603) -> ()
              }
              frame True {
              }
            }
            n2149 = property on="Trap Delta (MHz)" class="DigNum (strict)"("Val(Sgnl)"=w2598) -> ()  [unwired: 2 in, 2 out]
          }
          frame 2 {
            # "Wiggle"
            n2150 = Random Number (0-1)() -> (number: 0 to 1=w2609:dbl)
            n2151 = local read "Min TD"() -> (w2606:dbl)
            n2152 = local read "AF Time"() -> (w2614:u32)
            n2153 = Multiply(x=w2609, y="Wiggle TD") -> (x*y=w2607:dbl)
            n2154 = Tick Count (ms)() -> (millisecond timer value=w2615:u32)
            n2155 = Add(x=w2607, y=w2606) -> (x+y=w2604:dbl)
            n2156 = Subtract(x=w2615, y=w2614) -> (x-y=w2613:u32)
            n2157 = property on="Trap Delta (MHz)" class="DigNum (strict)"("Val(Sgnl)"=w2604) -> ()  [unwired: 2 in, 2 out]
            n2158 = Divide(x=w2613, y=u32 1000) -> (x/y=w2611:dbl)
            n2159 = Greater?(x=w2611, y="Wiggle time") -> (0:w2605:bool)
            n2160 = case shown="True" w2605 {
              frame False {
              }
              frame True {
                w2616 = u16 3 items=["Off", "Approach", "Wiggle", "Extend", "Tether Found"] ("Fish Status")
                n2161 = local write "Fish Status"(w2616) -> ()
              }
            }
          }
          frame 3 {
            # "Force"
            # "Extend"
            n2162 = local read "Trap Delta (MHz)"() -> (w2629:dbl)
            n2163 = Greater?(x=w2623, y="Extend Min F") -> (0:w2622:bool)
            n2164 = Add(x=w2629, y="Extend dTD") -> (x+y=w2627:dbl)
            n2165 = In Range and Coerce(upper limit="Max TD", x=w2627, lower limit=0.0) -> (coerced(x)=w2618:dbl, In Range?=w2617:bool)
            n2166 = Greater?(x=w2618, y="Extend Min TD") -> (0:w2621:bool)
            n2167 = And(x=w2621, y=w2622) -> (x .and. y?=w2620:bool)
            n2168 = case shown="False" w2620 {
              tunnel: w2617 -> [w2630 _]
              frame False {
                n2169 = case shown="True" w2630 {
                  frame False {
                    w2631 = u16 1 items=["Off", "Approach", "Wiggle", "Extend", "Tether Found"] ("Fish Status")
                    n2170 = local write "Fish Status"(w2631) -> ()
                  }
                  frame True {
                  }
                }
              }
              frame True {
                w2632 = u16 4 items=["Off", "Approach", "Wiggle", "Extend", "Tether Found"] ("Fish Status")
                n2171 = local write "Fish Status"(w2632) -> ()
              }
            }
            n2172 = property on="Trap Delta (MHz)" class="DigNum (strict)"("Val(Sgnl)"=w2618) -> ()  [unwired: 2 in, 2 out]
          }
          frame 4 {
            w2633 = u16 0 items=["Off", "Approach", "Wiggle", "Extend", "Tether Found"] ("Fish Status")
            n2173 = call <vilib>:"Beep.vi"("use system alert? (T)"=FALSE, "duration (msec)"=u32 100, "frequency (Hz)"=u32 466) -> ()  [unwired: 9 in]
            n2174 = local write "Fish Status"(w2633) -> ()
          }
        }
      }
      frame True {
        n2175 = case shown="Default" w2637 {
          frame 0 {
            w2639 = u16 1 items=["Off", "Approach", "Wiggle", "Extend", "Tether Found"] ("Fish Status")
            n2176 = local write "Fish Status"(w2639) -> ()
          }
          frame Default {
            w2640 = u16 0 items=["Off", "Approach", "Wiggle", "Extend", "Tether Found"] ("Fish Status")
            n2177 = local write "Fish Status"(w2640) -> ()
          }
        }
        n2178 = local write "Toggle AFish"(FALSE ("Toggle AFish")) -> ()
      }
    }
    n2179 = Bundle By Name(cluster=w2572, "Set 1"=w2571, "Set 2"=w2570) -> (w2568:cluster{"Set 1":dbl, "Set 2":dbl})
    n2180 = Divide(x=w2358, y=327.67) -> (x/y=→"Action (%)":dbl)
    n2181 = local read "Trap X (AI1)"() -> (w2378:T1)
    n2182 = Divide(x=w2568, y=3276.7) -> (x/y=w2567:cluster{"Set 1":dbl, "Set 2":dbl})
    n2183 = local write "AI2 (V)"(w2567) -> ()
    n2184 = Bundle(cluster=w2378, "Trap 1"=w2365, "Trap 2"=w2364) -> (→"Trap X (AI1)":T1)
    n2185 = Scale By Power Of 2(n=i16 12, x=ext 1.0) -> (x*2^n=w2260:ext)
    n2186 = Subtract(x=w2260, y=ext 1.0) -> (x-y=w2257:ext)
    n2187 = Divide(x=w2512, y=3276.7) -> (x/y=w2508:T49)
    n2188 = Multiply(x=w2264, y=ext 100.0) -> (x*y=w2258:ext)
    n2189 = Unbundle By Name(w2508) -> ("Green FB Ch 0"=w2511:dbl, "Green FB Ch 1"=w2510:dbl, "Green FB Ch 2"=w2509:dbl)
    n2190 = local read "All FB On/Off"() -> (w2248:bool)
    n2191 = Divide(x=w2258, y=w2257) -> (x/y=w2247:ext)
    "Trap 1 amplitude" <- w2247
    n2192 = Scale By Power Of 2(n=i16 12, x=ext 1.0) -> (x*2^n=w2253:ext)
    n2193 = Subtract(x=w2253, y=ext 1.0) -> (x-y=w2256:ext)
    n2194 = Multiply(x=w2249, y=ext 100.0) -> (x*y=w2255:ext)
    n2195 = Divide(x=w2511, y=w2509) -> (x/y=w2507:dbl)
    n2196 = Divide(x=w2510, y=w2509) -> (x/y=w2506:dbl)
    n2197 = flat-sequence "To save data" {
      tunnel: [w3669] -> w2592
      tunnel: [w3670] -> w2591
      tunnel: w2543 -> [w3663]
      tunnel: w2443 -> [w3667]
      tunnel: ["Save Calibration"] -> w2564
      tunnel: w2561 -> [w3666]
      tunnel: [w3659] -> w2560
      tunnel: [w3656] -> w2559
      tunnel: [w3653] -> w2558
      tunnel: w2542 -> [w3655]
      tunnel: w2455 -> [w3649]
      tunnel: [w3649] -> w2454
      tunnel: ["Start Saving"] -> w2421
      tunnel: [w3643] -> w2347
      tunnel: [w3642] -> w2346
      tunnel: w2592 -> [w3904]
      tunnel: w2591 -> [w3903]
      tunnel: w2348 -> [w3902]
      tunnel: w2564 -> [w3901]
      tunnel: w2560 -> [w3899]
      tunnel: w2559 -> [w3898]
      tunnel: w2558 -> [w3897]
      tunnel: w2430 -> [w3896]
      tunnel: w2464 -> [w3895]
      tunnel: w2454 -> [w3894]
      tunnel: w2421 -> [w3893]
      tunnel: w2419 -> [w3892]
      tunnel: w2395 -> [w3891]
      tunnel: w2347 -> [w3890]
      tunnel: w2346 -> [w3889]
      tunnel: w2345 -> [w3888]
      frame #0 {
        n2198 = Or(x="Save N Sets", y="Start Saving") -> (x .or. y?=w3650:bool)
        n2199 = To Double Precision Float(number=w3666) -> (double precision float=w3660:dbl)
        n2200 = Build Array(w3650, "Save Calibration", w3663, w3655) -> (w3665:bool[])
        n2201 = Compound Arithmetic op=OR("Save Calibration", w3663, w3650, w3655) -> (w3668:bool)
        n2202 = Boolean Array To Number(Boolean array=w3665) -> (number=w3662:u32)
        n2203 = feedback #19(FALSE ("Save APD Data\nwith Trap Data")) -> (w3644:bool)
        n2204 = feedback #20(refnum<k0> refnum) -> (w3671:refnum<file>)
        n2205 = feedback #21(refnum<k0> refnum) -> (w3646:refnum<file>)
        n2206 = feedback #22(FALSE ("Save APD Data\nwith Trap Data")) -> (w3654:bool)
        n2207 = feedback #23(refnum<k0> refnum) -> (w3657:refnum<file>)
        n2208 = feedback #24(0) -> (w3673:i32)
        n2209 = feedback #25() -> (w3661:u32)  [unwired: 1 out]
        n2210 = case shown="True" w3668 {
          tunnel: [w3680 1] -> w3669
          tunnel: w3673 -> [w3682 _]
          tunnel: [w3681 w3700] -> w3670
          tunnel: w3671 -> [w3681 _]
          tunnel: w3667 -> [_ w3720]
          tunnel: w3660 -> [_ w3718]
          tunnel: w3662 -> [_ w3721]
          tunnel: [w3679 w3699] -> w3659
          tunnel: w3661 -> [w3679 _]
          tunnel: [w3678 w3697] -> w3656
          tunnel: w3657 -> [w3678 _]
          tunnel: [w3677 w3696] -> w3653
          tunnel: w3654 -> [w3677 _]
          tunnel: "Start Saving" -> [_ w3694]
          tunnel: w3649 -> [_ w3693]
          tunnel: [w3676 w3684] -> w3642
          tunnel: w3646 -> [w3676 _]
          tunnel: [w3675 w3683] -> w3643
          tunnel: w3644 -> [w3675 _]
          frame False {
            n2211 = Increment(x=w3682) -> (x+1=w3680:i32)
          }
          frame True {
            w3690 = FALSE ("Start Saving")
            w3695 = 9.0  # File Version
            w3703 = FALSE ("prepend array or string size? (T)")
            w3701 = T30."big-endian, network order" ("byte order (0:big-endian, network order)")
            # "write file headers"
            n2212 = local read "BD 1 Frequency 1 (MHz)"() -> (w3717:dbl)
            n2213 = local read "BD 2 Frequency 1 (MHz)"() -> (w3716:dbl)
            n2214 = local read "BD 1 Frequency 2 (MHz)"() -> (w3715:dbl)
            n2215 = local read "BD 2 Frequency 2 (MHz)"() -> (w3714:dbl)
            n2216 = local read "BD 1 Frequency 3 (MHz)"() -> (w3713:dbl)
            n2217 = local read "BD 2 Frequency 3 (MHz)"() -> (w3712:dbl)
            n2218 = Array Size(array=w3693) -> (size(s)=w3692:i32)
            n2219 = To Double Precision Float(number=w3692) -> (double precision float=w3691:dbl)
            n2220 = local write "Save Calibration"(w3690) -> ()
            n2221 = local write "Start Saving"(w3690) -> ()
            n2222 = Build Array("Save APD Data\nwith Trap Data", "Save Trap Pos. Data") -> (w3687:bool[])
            n2223 = Boolean Array To Number(Boolean array=w3687) -> (number=w3686:u32)
            n2224 = Build Array(w3717, w3716, w3715, w3714, w3713, w3712) -> (w3711:dbl[])
            n2225 = case shown="2" w3721 {
              tunnel: w3720 -> [w3792 w3812 w3828 w3866]
              tunnel: w3691 -> [w3797 w3819 w3848 w3885]
              tunnel: w3718 -> [w3796 w3818 w3847 w3884]
              tunnel: [w3793 w3814 w3839 w3876] -> w3709
              tunnel: [w3784 "Cal sets to save" w3829 w3867] -> w3699
              tunnel: w3711 -> [w3794 w3815 w3841 w3878]
              tunnel: "Save APD Data\nwith Trap Data" -> [w3791 _ w3825 w3864]
              tunnel: [w3791 w3806 w3825 w3864] -> w3696
              tunnel: w3695 -> [w3787 w3807 w3823 w3862]
              tunnel: w3694 -> [w3786 _ _ _]
              tunnel: [w3777 w3806 w3822 w3852] -> w3683
              tunnel: "Save Trap Pos. Data" -> [w3777 _ w3822 w3852]
              tunnel: w3686 -> [w3776 _ w3821 w3851]
              frame 1, Default {
                # "timeseries"
                n2226 = case shown="True" "Profile" {
                  tunnel: [w3800 w3803] -> w3781
                  tunnel: [w3800 w3802] -> w3780
                  tunnel: [w3800 w3801] -> w3779
                  tunnel: [w3800 w3805] -> w3778
                  frame False {
                    w3800 = 0.0 ("f")
                  }
                  frame True {
                    n2227 = local read "Current Position"() -> (w3804:dbl[])
                    n2228 = local read "Y change (mm)"() -> (w3805:dbl)
                    n2229 = call "subVI_explode3array.vi"("Array"=w3804) -> ("x"=w3803:dbl, "y"=w3802:dbl, "z"=w3801:dbl)  [unwired: 12 in]
                  }
                }
                n2230 = local read "Save ave N"() -> (w3799:dbl)
                n2231 = Multiply(x=w3799, y=w3792) -> (x*y=w3798:dbl)
                n2232 = To Double Precision Float(number=w3776) -> (double precision float=w3790:dbl)
                n2233 = Build Array(w3787, w3792, w3798, w3797, w3796, 0.0 ("f")) -> (w3795:dbl[])
                n2234 = Build Array(w3790, w3781, w3780, w3779, w3778) -> (w3788:dbl[])
                n2235 = Select(t=u32 4000000000, s=w3786, f="N sets to save") -> (s? t:f=w3784:u32)
                n2236 = Build Array (concatenate)(w3795, w3794, w3788) -> (w3793:dbl[])
              }
              frame 2 {
                w3809 = 0.0 ("f")
                w3806 = FALSE ("Save APD Data\nwith Trap Data")
                # "calibration"
                n2237 = Boolean To (0,1)(Boolean=w3806) -> (0, 1=w3811:i16)
                n2238 = To Double Precision Float(number=w3811) -> (double precision float=w3810:dbl)
                n2239 = Build Array(w3810, w3809, w3809, w3809, w3809) -> (w3808:dbl[])
                n2240 = Build Array(w3807, w3812, w3812, w3819, w3818, 1.0 ("t")) -> (w3816:dbl[])
                n2241 = Build Array (concatenate)(w3816, w3815, w3808) -> (w3814:dbl[])
                "Calibrating Trap..." <- TRUE ("Calibrating...")
              }
              frame 4 {
                w3826 = 0.0 ("f")
                # "write file header for a trap \nraster scan"
                # "scan dir (x/y = 0/1)"
                # "cycles/step"
                # "n scans (f/b)"
                # "steps"
                # "freq. range"
                # "AOD raster scan"
                n2242 = local read "Number of F/B Scans (AOD)"() -> (w3833:u16)
                n2243 = local read "Cycles/step (AOD)"() -> (w3835:u64)
                n2244 = local read "Scan Range (MHz)"() -> (w3838:dbl)
                n2245 = local read "Scan steps (AOD)"() -> (w3837:u64)
                n2246 = local read "Scan BD"() -> (w3845:bool)
                n2247 = local read "Save ave N"() -> (w3850:dbl)
                n2248 = Boolean To (0,1)(Boolean=w3845) -> (0, 1=w3844:i16)
                n2249 = To Double Precision Float(number=w3833) -> (double precision float=w3832:dbl)
                n2250 = To Double Precision Float(number=w3837) -> (double precision float=w3836:dbl)
                n2251 = To Double Precision Float(number=w3835) -> (double precision float=w3834:dbl)
                n2252 = To Double Precision Float(number=w3844) -> (double precision float=w3843:dbl)
                n2253 = Multiply(x=w3850, y=w3828) -> (x*y=w3849:dbl)
                n2254 = To Double Precision Float(number=w3821) -> (double precision float=w3827:dbl)
                n2255 = Build Array(w3827, w3826, w3826, w3826, w3826) -> (w3824:dbl[])
                n2256 = local read "N sets should be saved"() -> (w3830:dbl)
                n2257 = Build Array(w3843, w3838, w3836, w3834, w3832) -> (w3840:dbl[])
                n2258 = Build Array(w3823, w3828, w3849, w3848, w3847, 2.0 ("t")) -> (w3842:dbl[])
                n2259 = Round Toward +Infinity(x=w3830) -> (ceil(x): smallest int >= x=w3831:dbl)
                n2260 = Build Array (concatenate)(w3842, w3841, w3824, w3840) -> (w3839:dbl[])
                n2261 = To Unsigned Long Integer(number=w3831) -> (unsigned 32bit integer=w3829:u32)
              }
              frame 8 {
                w3859 = 0.0 ("f")
                # "MCL raster scan"
                n2262 = local read "Number of scans (MCL)"() -> (w3854:u64)
                n2263 = local read "Scan lines (y)"() -> (w3853:u64)
                n2264 = local read "2D or 1D Scan"() -> (w3856:bool)
                n2265 = local read "Scan Range (V)\n(of steps)"() -> (w3875:dbl)
                n2266 = local read "Fast Scan Dir"() -> (w3882:bool)
                n2267 = local read "Cycles/step (MCL)"() -> (w3872:u64)
                n2268 = local read "Scan steps (MCL)"() -> (w3874:u64)
                n2269 = Select(t=w3853, s=w3856, f=w3854) -> (s? t:f=w3855:u64)
                n2270 = Boolean To (0,1)(Boolean=w3856) -> (0, 1=w3858:i16)
                n2271 = local read "Save ave N"() -> (w3887:dbl)
                n2272 = local read "Initial X"() -> (w3861:dbl)
                n2273 = local read "Initial Y"() -> (w3860:dbl)
                n2274 = To Double Precision Float(number=w3858) -> (double precision float=w3857:dbl)
                n2275 = Boolean To (0,1)(Boolean=w3882) -> (0, 1=w3881:i16)
                n2276 = To Double Precision Float(number=w3855) -> (double precision float=w3870:dbl)
                n2277 = To Double Precision Float(number=w3874) -> (double precision float=w3873:dbl)
                n2278 = To Double Precision Float(number=w3872) -> (double precision float=w3871:dbl)
                n2279 = To Double Precision Float(number=w3881) -> (double precision float=w3880:dbl)
                n2280 = Multiply(x=w3887, y=w3866) -> (x*y=w3886:dbl)
                n2281 = To Double Precision Float(number=w3851) -> (double precision float=w3865:dbl)
                n2282 = local read "N sets should be saved (MCL)"() -> (w3868:dbl)
                n2283 = Build Array(w3865, w3857, w3859, w3859, w3859) -> (w3863:dbl[])
                n2284 = Build Array(w3880, w3875, w3873, w3871, w3870, w3861, w3860) -> (w3877:dbl[])
                n2285 = Build Array(w3862, w3866, w3886, w3885, w3884, 3.0 ("t")) -> (w3879:dbl[])
                n2286 = Round Toward +Infinity(x=w3868) -> (ceil(x): smallest int >= x=w3869:dbl)
                n2287 = Build Array (concatenate)(w3879, w3878, w3863, w3877) -> (w3876:dbl[])
                n2288 = To Unsigned Long Integer(number=w3869) -> (unsigned 32bit integer=w3867:u32)
              }
            }
            n2289 = local read "Index"() -> (w3726:dbl)
            n2290 = call "Create new save file.vi"("Insert"="", "Ext"=".dat", "Index In"=w3726) -> ("Path Out"=w3685:path, "Index Out"=w3698:dbl)
            n2291 = local write "Save file name"(w3685) -> ()
            n2292 = local write "Index"(w3698) -> ()
            n2293 = local write "Save index"(w3698) -> ()
            n2294 = Array Size(array=w3709) -> (size(s)=w3710:i32)
            n2295 = Open/Create/Replace File(file path (use dialog)=w3685, operation (0:open)=T24."create", access (0:read/write)=enum16{"read/write", "read-only", "write-only"}."write-only") -> (refnum out=w3723:refnum<file>)  [unwired: 1 in, 4 out]
            n2296 = local write "Saving..."(TRUE ("Saving...")) -> ()
            n2297 = To Double Precision Float(number=w3710) -> (double precision float=w3708:dbl)
            n2298 = String Length(string="Comment (data description)") -> (length=w3706:i32)
            n2299 = To Double Precision Float(number=w3706) -> (double precision float=w3705:dbl)
            n2300 = Deny Access(7:w3723) -> (3:w3722:refnum<file>)  [unwired: 1 in, 2 out]
            n2301 = Build Array (concatenate)(w3708, w3709, w3705) -> (w3707:dbl[])
            n2302 = case "If fluorescence data to be saved" shown="True" w3696 {
              tunnel: w3685 -> [_ w3775]
              tunnel: [refnum<k0> refnum w3755] -> w3697
              frame False {
              }
              frame True {
                w3754 = 0.0
                n2303 = local read "APD Integration Time (s)"() -> (w3760:dbl)
                n2304 = local read "N APD Samp/step"() -> (w3753:dbl)
                n2305 = Path To String(path=w3775) -> (string=w3774:string)
                n2306 = String Length(string=w3774) -> (length=w3773:i32)
                n2307 = Subtract(x=w3773, y=4) -> (x-y=w3771:i32)
                n2308 = String Subset(string=w3774, length (rest)=w3771) -> (substring=w3770:string)  [unwired: 1 out]
                n2309 = Build Array(w3760, w3753, w3754, w3754, w3754, w3754, w3754, w3754) -> (w3757:dbl[])
                n2310 = Concatenate Strings(w3770, "_fl.dat" ("string")) -> (w3768:string)
                n2311 = Array Size(array=w3757) -> (size(s)=w3759:i32)
                n2312 = String To Path(string=w3768) -> (path=w3764:path)
                n2313 = Open/Create/Replace File(file path (use dialog)=w3764, operation (0:open)=T24."create", access (0:read/write)=enum16{"read/write", "read-only", "write-only"}."write-only") -> (refnum out=w3765:refnum<file>)  [unwired: 1 in, 4 out]
                n2314 = Deny Access(7:w3765) -> (3:w3761:refnum<file>)  [unwired: 1 in, 2 out]
                n2315 = To Double Precision Float(number=w3759) -> (double precision float=w3758:dbl)
                n2316 = Build Array (concatenate)(w3758, w3757) -> (w3756:dbl[])
                n2317 = Write to Binary File(file (use dialog)=w3761, data=w3756, 5:FALSE ("prepend array or string size? (T)"), 9:T30."big-endian, network order" ("byte order (0:big-endian, network order)")) -> (refnum out=w3755:refnum<file>)  [unwired: 1 in, 3 out]
              }
            }
            n2318 = case shown="True" w3683 {
              tunnel: w3685 -> [_ w3737]
              tunnel: [refnum<k0> refnum w3736] -> w3684
              frame False {
              }
              frame True {
                w3732 = 0.0 ("element")
                n2319 = Path To String(path=w3737) -> (string=w3751:string)
                n2320 = Build Array(w3732, w3732, w3732, w3732, w3732, w3732, w3732, w3732) -> (w3733:dbl[])
                n2321 = String Length(string=w3751) -> (length=w3750:i32)
                n2322 = Subtract(x=w3750, y=4) -> (x-y=w3748:i32)
                n2323 = Array Size(array=w3733) -> (size(s)=w3735:i32)
                n2324 = String Subset(string=w3751, length (rest)=w3748) -> (substring=w3747:string)  [unwired: 1 out]
                n2325 = To Double Precision Float(number=w3735) -> (double precision float=w3734:dbl)
                n2326 = Concatenate Strings(w3747, "_pos.dat" ("string")) -> (w3745:string)
                n2327 = Build Array (concatenate)(w3734, w3733) -> (w3731:dbl[])
                n2328 = String To Path(string=w3745) -> (path=w3741:path)
                n2329 = Open/Create/Replace File(file path (use dialog)=w3741, operation (0:open)=T24."create", access (0:read/write)=enum16{"read/write", "read-only", "write-only"}."write-only") -> (refnum out=w3742:refnum<file>)  [unwired: 1 in, 4 out]
                n2330 = Deny Access(7:w3742) -> (3:w3738:refnum<file>)  [unwired: 1 in, 2 out]
                n2331 = Write to Binary File(file (use dialog)=w3738, data=w3731, 5:FALSE ("prepend array or string size? (T)"), 9:T30."big-endian, network order" ("byte order (0:big-endian, network order)")) -> (refnum out=w3736:refnum<file>)  [unwired: 1 in, 3 out]
              }
            }
            n2332 = Write to Binary File(file (use dialog)=w3722, data=w3707, 5:w3703, 9:w3701) -> (refnum out=w3704:refnum<file>)  [unwired: 1 in, 3 out]
            n2333 = Write to Binary File(file (use dialog)=w3704, data="Comment (data description)", 5:w3703, 9:w3701) -> (refnum out=w3700:refnum<file>)  [unwired: 1 in, 3 out]
          }
        }
        n2334 = feedback-in #19(w3643) -> ()
        n2335 = feedback-in #20(w3670) -> ()
        n2336 = feedback-in #21(w3642) -> ()
        n2337 = feedback-in #22(w3653) -> ()
        n2338 = feedback-in #23(w3656) -> ()
        n2339 = feedback-in #24(w3669) -> ()
        n2340 = feedback-in #25(w3659) -> ()
      }
      frame #1 {
        n2341 = local read "Saving..."() -> (w3900:bool)
        n2342 = case shown="True" w3900 {
          tunnel: w3904 -> [_ w3914]
          tunnel: w3903 -> [_ w3928]
          tunnel: w3902 -> [_ w3924]
          tunnel: w3901 -> [_ w3923]
          tunnel: w3899 -> [_ w3922]
          tunnel: w3898 -> [_ w3917]
